vi "Write Class Type.vi"(8 "error in (no error)":errorcluster, 10 "domain class type":T1 items=["Domain"=0, "Domain_Steady"=100, "Domain_Steady_2D_Rect"=121, "Domain_Steady_2D_Polygon"=122, "Domain_Evolut"=200, "Domain_Evolut_1D"=210, "Domain_Evolut_2D_Rect"=221], 11 "Domain.lvclass in":refnum<class "NI_Domain.lvclass">) -> (0 "error out":errorcluster, 3 "Domain.lvclass out":refnum<class "NI_Domain.lvclass">)   [LabVIEW 2017, in "NI_PDE.lvlib" / "NI_Domain.lvclass"]
uses:
  <vilib>/gmath/pde.llb/DomainClass/NI_Domain.lvclass
  <vilib>/gmath/pde.llb/DomainClass/Class Type.ctl
  <vilib>/gmath/pde.llb/DomainClass/NI_Domain.lvclass/NI_Domain.ctl
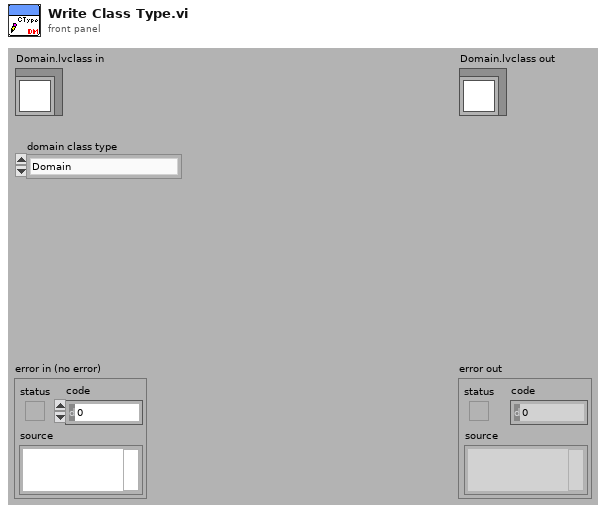
[diagram p1: front panel]
types:
  T1 = typedef "NI_PDE.lvlib/NI_Domain.lvclass/Class Type.ctl" = i32
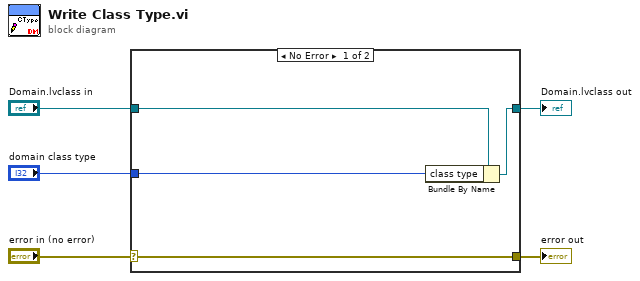
[diagram p0: block diagram]
diagram:
  n1 = case shown="No Error" "error in (no error)" {
    selector: "error in (no error)" -> [w9 w10]
    tunnel: [w9 w10] -> w4
    tunnel: [w7 w11] -> w2
    tunnel: "Domain.lvclass in" -> [w8 w11]
    tunnel: "domain class type" -> [w6 _]
    frame No Error {
      n2 = Bundle By Name(cluster=w8, "class type"=w6) -> (w7:refnum<class "NI_Domain.lvclass">)
    }
    frame Error {
    }
  }
  "error out" <- w4
  "Domain.lvclass out" <- w2
